vi "dfd_Check Group Delay Design Specs.vi"(6 "fs [Hz]":dbl=1.0 format="%.2f", 8 "error in (no error)":errorcluster, 10 "freq range":cluster{"f lo":dbl, "f hi":dbl}={"f lo"=0.0, "f hi"=0.1}, 11 "filter in":T1={"mSRate_Fs"=1.0, "mSRate_Version"="1.0", "mSRate_Comments"="", "mSRate_OrgCoef"={"type"=enum."Undefined", "gain"=1.0, "coef a (k)"=[], "coef b (v)"=[]}, "mSRate_CurCoef"={"type"=enum."Undefined", "gain"=1.0, "coef a (k)"=[], "coef b (v)"=[]}, "mSRate_Quantized?"=FALSE, "mSRate_QCoef"={"type"=enum."Undefined", "gain"=1.0, "coef a (k)"=[], "coef b (v)"=[]}, "mSRate_QSettings"=[], "mSRate_Order"=0, "mSRate_Scaling"={"mSRate_ScaleByPowerOf2?"=FALSE, "mSRate_ScaleType"=enum."No Norm"}} {"mSRate_QSettings"."source" items=["Coef a/k"=0, "Coef b/v"=7, "Input"=1, "Output"=2, "Multiplicand"=3, "Product"=4, "Sum"=5, "Delay"=6, "Gain"=8]}) -> (0 "error IO":errorcluster, 2 "dup freq range":cluster{"f lo":dbl, "f hi":dbl}={"f lo"=0.0, "f hi"=0.1}, 3 "dup filter in":T1={"mSRate_Fs"=1.0, "mSRate_Version"="1.0", "mSRate_Comments"="", "mSRate_OrgCoef"={"type"=enum."Undefined", "gain"=1.0, "coef a (k)"=[], "coef b (v)"=[]}, "mSRate_CurCoef"={"type"=enum."Undefined", "gain"=1.0, "coef a (k)"=[], "coef b (v)"=[]}, "mSRate_Quantized?"=FALSE, "mSRate_QCoef"={"type"=enum."Undefined", "gain"=1.0, "coef a (k)"=[], "coef b (v)"=[]}, "mSRate_QSettings"=[], "mSRate_Order"=0, "mSRate_Scaling"={"mSRate_ScaleByPowerOf2?"=FALSE, "mSRate_ScaleType"=enum."No Norm"}} {"mSRate_QSettings"."source" items=["Coef a/k"=0, "Coef b/v"=7, "Input"=1, "Output"=2, "Multiplicand"=3, "Product"=4, "Sum"=5, "Delay"=6, "Gain"=8]}, 4 "dup fs [Hz]":dbl=1.0 format="%.2f")   [LabVIEW 2017, in "NI_DigFilter_Design.lvlib"]
uses:
  <vilib>/addons/Digital Filter Design/NI_DigFilter_Design.lvlib
  <vilib>/addons/Digital Filter Design/_Objects.llb/DFD Filter Obj.ctl
  <vilib>/addons/Digital Filter Design/_Objects.llb/DFD Filter Coef.ctl
  <vilib>/addons/Digital Filter Design/_Objects.llb/DFD Filter Structure Type Selector.ctl
  <vilib>/addons/Digital Filter Design/_Objects.llb/dfd_Internal Quantization Settings.ctl
  <vilib>/addons/Digital Filter Design/_Objects.llb/dfd_Internal Quantization Srcs.ctl
  <vilib>/addons/Digital Filter Design/_Objects.llb/DFD Coef Norm Type.ctl
  <vilib>/addons/Digital Filter Design/NI_DigFilterLicensed.lvlib
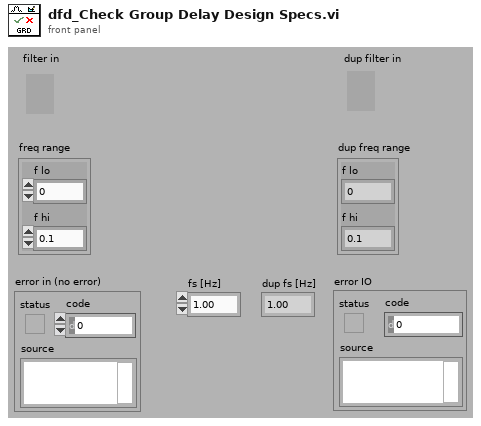
[diagram p1: front panel]
types:
  T1 = typedef "NI_DigFilterLicensed.lvlib/DFD Filter Obj.ctl" = cluster{"mSRate_Fs":dbl, "mSRate_Version":string, "mSRate_Comments":string, "mSRate_OrgCoef":T2, "mSRate_CurCoef":T2, "mSRate_Quantized?":bool, "mSRate_QCoef":T2, "mSRate_QSettings":T4[], "mSRate_Order":i32, "mSRate_Scaling":cluster{"mSRate_ScaleByPowerOf2?":bool, "mSRate_ScaleType":T6}}
  T2 = typedef "NI_DigFilterLicensed.lvlib/DFD Filter Coef.ctl" = cluster{"type":T3, "gain":dbl, "coef a (k)":dbl[], "coef b (v)":dbl[]}
  T3 = typedef "NI_DigFilterLicensed.lvlib/DFD Filter Structure Type Selector.ctl" = enum16{"Undefined", "FIR Direct Form", "FIR Direct Form Transposed", "FIR Symmetric", "FIR Antisymmetric", "IIR Direct Form I", "IIR Direct Form I Transposed", "IIR Direct Form II", "IIR Direct Form II Transposed", "IIR Cascaded Second Order Sections Form I", "IIR Cascaded Second Order Sections Form I Transposed", "IIR Cascaded Second Order Sections Form II", "IIR Cascaded Second Order Sections Form II Transposed", "Lattice Allpass (basic sections)", "Lattice Allpass (one multiplier sections)", "Lattice Allpass (normalized sections)", "Lattice AR (basic sections)", "Lattice AR (one multiplier sections)", "Lattice AR (normalized sections)", "Lattice MA (minimum phase)", "Lattice MA (maximum phase)", "Lattice ARMA (basic sections)", "Lattice ARMA (one multiplier sections)", "Lattice ARMA (normalized sections)"}
  T4 = typedef "NI_DigFilterLicensed.lvlib/dfd_Internal Quantization Settings.ctl" = cluster{"source":T5, "wl":i16, "iwl":i16, "overflow mode":enum16{"Saturation", "Wrap"}, "rounding mode":enum16{"Nearest", "Truncation"}, "signed?":bool}
  T5 = typedef "NI_DigFilterLicensed.lvlib/dfd_Internal Quantization Srcs.ctl" = u16
  T6 = typedef "NI_DigFilterLicensed.lvlib/DFD Coef Norm Type.ctl" = enum16{"No Norm", "Time Domain 1-Norm", "Time Domain 2-Norm", "Time Domain Inf-Norm"}
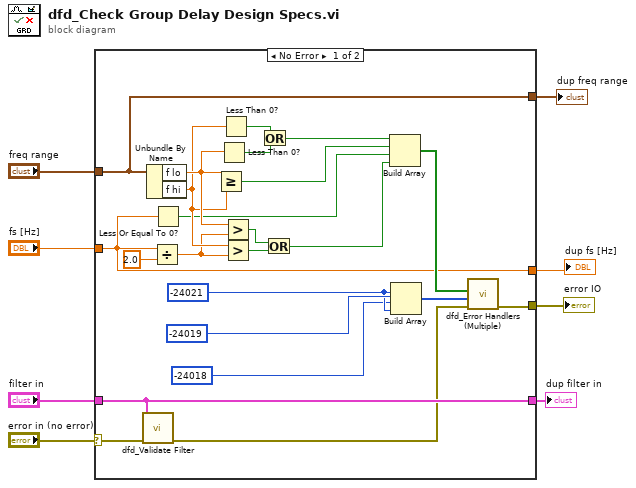
[diagram p0: block diagram]
diagram:
  n1 = case shown="No Error" "error in (no error)" {
    selector: "error in (no error)" -> [w15 w32]
    tunnel: [w20 w32] -> w7
    tunnel: "fs [Hz]" -> [w16 _]
    tunnel: "freq range" -> [w17 _]
    tunnel: [w17 _] -> w4
    tunnel: [w16 _] -> w3
    tunnel: "filter in" -> [w14 _]
    tunnel: [w14 _] -> w1
    frame No Error {
      w10 = -24021 ("ERR_FREQ_RANGE_WRONG")
      n2 = call <vilib>:"dfd_Validate Filter.vi"("error in (no error)"=w15, "filter in"=w14) -> ("error out"=w13:errorcluster)  [unwired: 1 in, 8 out]
      n3 = Unbundle By Name(w17) -> ("f lo"=w28:dbl, "f hi"=w27:dbl)
      n4 = Divide(x=w16, y=2.0) -> (x/y=w26:dbl)
      n5 = Less Or Equal To 0?(x=w16) -> (x <= 0?=w11:bool)
      n6 = Greater Or Equal?(x=w28, y=w27) -> (x >= y?=w21:bool)
      n7 = Less Than 0?(x=w28) -> (x < 0?=w30:bool)
      n8 = Less Than 0?(x=w27) -> (x < 0?=w31:bool)
      n9 = Greater?(x=w28, y=w26) -> (0:w25:bool)
      n10 = Greater?(x=w27, y=w26) -> (0:w24:bool)
      n11 = Or(x=w31, y=w30) -> (x .or. y?=w22:bool)
      n12 = Or(x=w25, y=w24) -> (x .or. y?=w12:bool)
      n13 = Build Array(w22, w21, w11, w12) -> (w18:bool[])
      n14 = Build Array(w10, -24019 ("ERR_FREQ_NOT_ASCENDING"), -24018 ("ERR_FS_LE_ZERO"), w10) -> (w19:i32[])
      n15 = call <vilib>:"dfd_Error Handlers (Multiple).vi"("error in (no error)"=w13, "error sources"=w19, "condition failed?"=w18) -> ("error out"=w20:errorcluster)  [unwired: 8 out]
    }
    frame Error {
    }
  }
  "error IO" <- w7
  "dup freq range" <- w4
  "dup fs [Hz]" <- w3
  "dup filter in" <- w1
